vi "ScopeConfigure.vi"(0 "VISA resource name":refnum<visa-resource-name>, 1 "scaleTime":dbl format="%#_6f", 2 "Channel 0/1":i32, 3 "Single Capture":bool, 4 "scaleVoltage":dbl, 5 "error in (no error)":errorcluster, 6 "Channel (0: Channel 1)":u16(ring) items=["Channel 1", "Channel 2", "Channel 3", "Channel 4"], 7 "Attenuation":i32, 10 "Vertical Coupling (0: DC)":u16(ring) items=["DC", "AC", "Ground"], 11 "Trigger Type (0: Edge)":u16(ring) items=["Edge", "Pulse", "Video", "Pattern", "Duration"], 12 "BW Selector":bool, 13 "Trigger Level":dbl) -> (14 "VISA resource name out":refnum<visa-resource-name>, 19 "error out":errorcluster)   [LabVIEW 2018]
panel:
  out "concatenated string":string
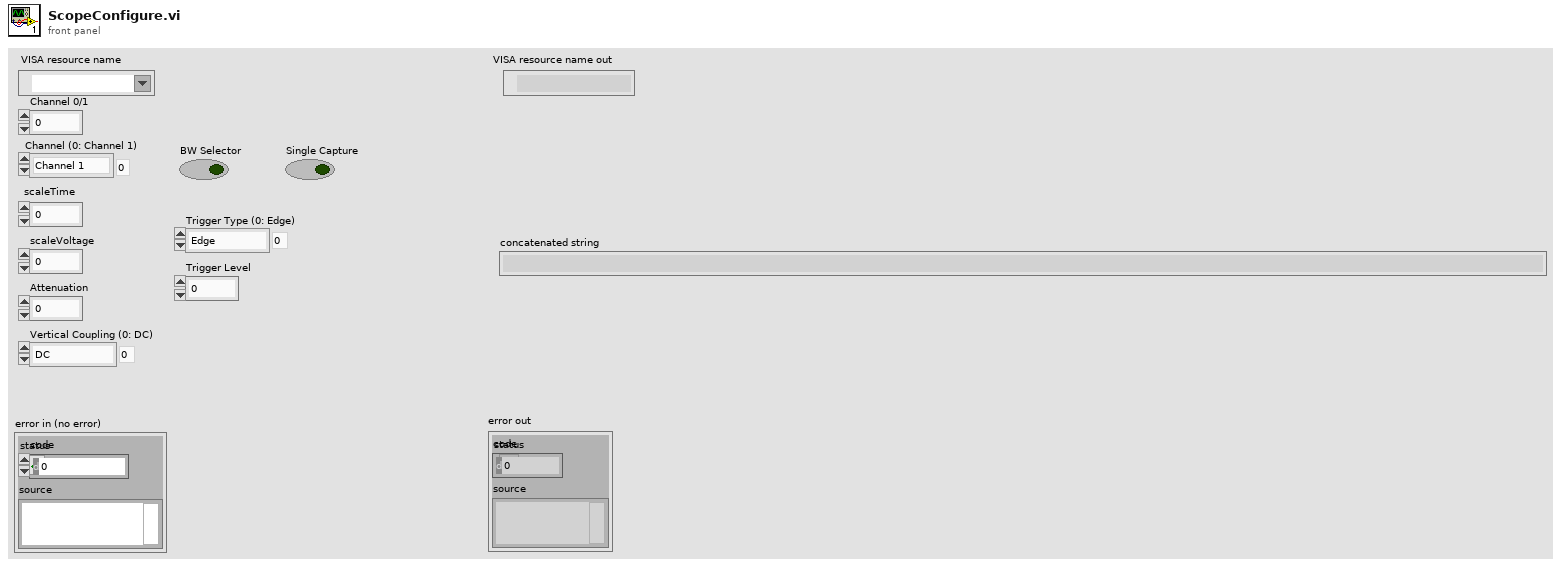
[diagram p1: front panel]
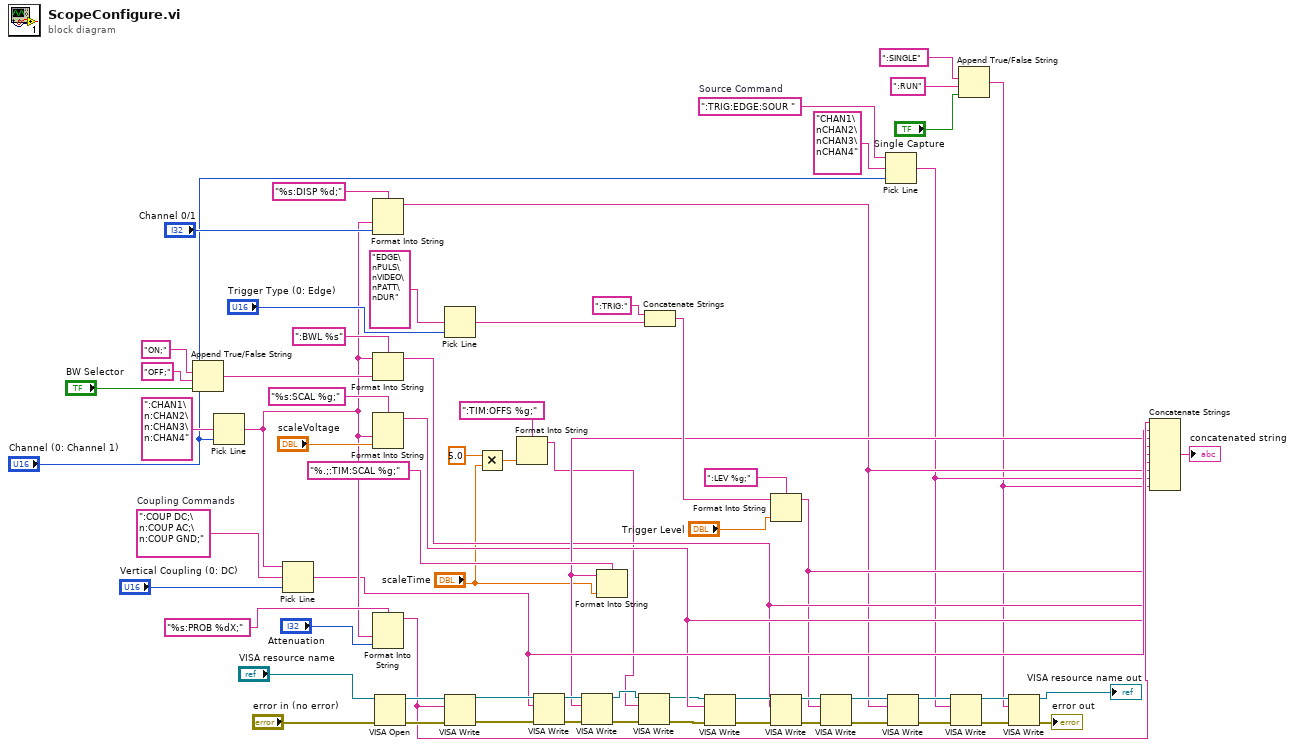
[diagram p0: block diagram]
diagram:
  w22 = ":TRIG:EDGE:SOUR "  # Source Command
  w61 = ":COUP DC;\n:COUP AC;\n:COUP GND;"  # Coupling Commands
  n1 = Append True/False String(1:"BW Selector", 2:"OFF;" ("false string"), 3:"ON;" ("true string")) -> (0:w58:string)  [unwired: 1 out]
  n2 = Pick Line(multi-line string=":CHAN1\n:CHAN2\n:CHAN3\n:CHAN4" ("多行字符串"), line index="Channel (0: Channel 1)") -> (output string=w29:string)  [unwired: 1 out]
  n3 = Pick Line(string ("")=w29, multi-line string=w61, line index="Vertical Coupling (0: DC)") -> (output string=w20:string)
  n4 = Format Into String(format string="%s:DISP %d;", w29, "Channel 0/1") -> (resulting string=w15:string)  [unwired: 2 in, 1 out]
  n5 = Format Into String(format string=":BWL %s", initial string=w29, w58) -> (resulting string=w17:string)  [unwired: 1 in, 1 out]
  n6 = Format Into String(format string="%s:SCAL %g;", w29, "scaleVoltage") -> (resulting string=w18:string)  [unwired: 2 in, 1 out]
  n7 = Format Into String(format string="%s:PROB %dX;", w29, "Attenuation") -> (resulting string=w21:string)  [unwired: 2 in, 1 out]
  n8 = VISA Open(error in (no error)="error in (no error)", VISA resource name="VISA resource name") -> (VISA resource name=w37:refnum<visa-resource-name>, error out=w38:errorcluster)  [unwired: 3 in]
  n9 = Pick Line(multi-line string="EDGE\nPULS\nVIDEO\nPATT\nDUR", line index="Trigger Type (0: Edge)") -> (output string=w54:string)  [unwired: 1 out]
  n10 = VISA Write(VISA resource name=w37, write buffer=w21, error in (no error)=w38) -> (VISA resource name out=w42:refnum<visa-resource-name>, error out=w43:errorcluster)  [unwired: 1 out]
  n11 = Multiply(x=5.0, y="scaleTime") -> (x*y=w3:dbl)
  n12 = Format Into String(format string=":TIM:OFFS %g;", w3) -> (resulting string=w5:string)  [unwired: 2 in, 1 out]
  n13 = VISA Write(VISA resource name=w42, write buffer=w20, error in (no error)=w43) -> (VISA resource name out=w41:refnum<visa-resource-name>, error out=w44:errorcluster)  [unwired: 1 out]
  n14 = Format Into String(format string="%.;:TIM:SCAL %g;", "scaleTime") -> (resulting string=w19:string)  [unwired: 2 in, 1 out]
  n15 = VISA Write(VISA resource name=w41, write buffer=w19, error in (no error)=w44) -> (VISA resource name out=w6:refnum<visa-resource-name>, error out=w45:errorcluster)  [unwired: 1 out]
  n16 = VISA Write(VISA resource name=w6, write buffer=w5, error in (no error)=w45) -> (VISA resource name out=w7:refnum<visa-resource-name>, error out=w8:errorcluster)  [unwired: 1 out]
  n17 = Concatenate Strings(":TRIG:" ("string (\"\")"), w54) -> (w48:string)
  n18 = VISA Write(VISA resource name=w7, write buffer=w18, error in (no error)=w8) -> (VISA resource name out=w40:refnum<visa-resource-name>, error out=w46:errorcluster)  [unwired: 1 out]
  n19 = Format Into String(format string=":LEV %g;", initial string=w48, "Trigger Level") -> (resulting string=w16:string)  [unwired: 1 in, 1 out]
  n20 = VISA Write(VISA resource name=w40, write buffer=w17, error in (no error)=w46) -> (VISA resource name out=w39:refnum<visa-resource-name>, error out=w47:errorcluster)  [unwired: 1 out]
  n21 = VISA Write(VISA resource name=w39, write buffer=w16, error in (no error)=w47) -> (VISA resource name out=w32:refnum<visa-resource-name>, error out=w34:errorcluster)  [unwired: 1 out]
  n22 = Pick Line(string ("")=w22, multi-line string="CHAN1\nCHAN2\nCHAN3\nCHAN4" ("多行字符串"), line index="Channel (0: Channel 1)") -> (output string=w14:string)
  n23 = VISA Write(VISA resource name=w32, write buffer=w15, error in (no error)=w34) -> (VISA resource name out=w25:refnum<visa-resource-name>, error out=w26:errorcluster)  [unwired: 1 out]
  n24 = VISA Write(VISA resource name=w25, write buffer=w14, error in (no error)=w26) -> (VISA resource name out=w24:refnum<visa-resource-name>, error out=w23:errorcluster)  [unwired: 1 out]
  n25 = Append True/False String(1:"Single Capture", 2:":RUN" ("false string"), 3:":SINGLE") -> (0:w10:string)  [unwired: 1 out]
  n26 = VISA Write(VISA resource name=w24, write buffer=w10, error in (no error)=w23) -> (VISA resource name out=→"VISA resource name out":refnum<visa-resource-name>, error out=→"error out":errorcluster)  [unwired: 1 out]
  n27 = Concatenate Strings(w21, w20, w19, w18, w17, w16, w15, w14, w10) -> (→"concatenated string":string)
